vi "zadanie_1.vi"() -> ()   [LabVIEW 2020]
panel:
  in  "wartosc do wpisania":dbl
  in  "stop":bool
  out "wartosc komorki":dbl
  in  "Boolean 2":bool
  out "Boolean":bool
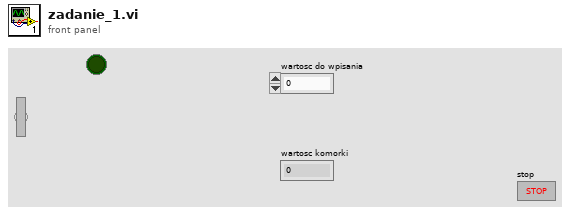
[diagram p1: front panel]
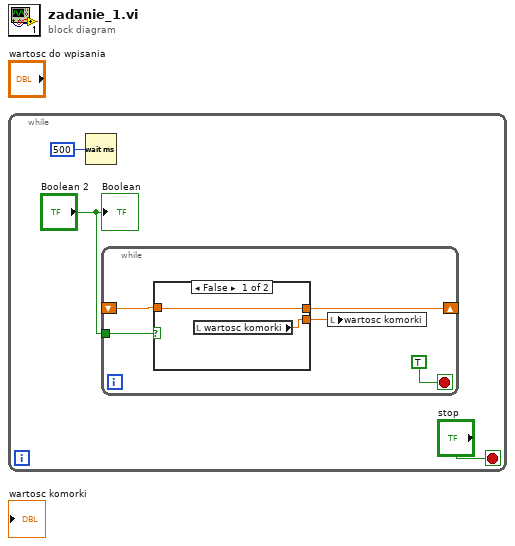
[diagram p0: block diagram]
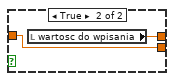
[diagram p2: hidden frame]
diagram:
  n1 = while {
    stop <- "stop" stop-if-true
    n2 = Wait (ms)(milliseconds to wait=u32 500) -> ()  [unwired: 1 out]
    n3 = while {
      tunnel: "Boolean 2" -> [w8]
      shift-right: [w6] -> _
      shift-left: _ -> [w5]
      stop <- TRUE stop-if-true
      n4 = case shown="False" w8 {
        tunnel: [w9 w11] -> w6
        tunnel: w5 -> [w9 w12]
        tunnel: [w10 w12] -> w4
        frame False {
          n5 = local read "wartosc komorki"() -> (w10:dbl)
        }
        frame True {
          n6 = local read "wartosc do wpisania"() -> (w11:dbl)
        }
      }
      n7 = local write "wartosc komorki"(w4) -> ()
    }
    "Boolean" <- "Boolean 2"
  }
